vi "Ray2p0andDir.vi"(10 "Ray":T1) -> (2 "Dir":dbl[](array[numeric]), 3 "P0":dbl[](array[numeric]))   [LabVIEW 2014]
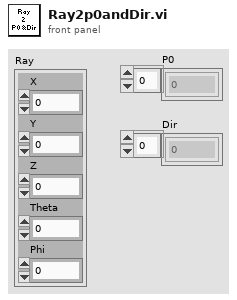
[diagram p1: front panel]
types:
  T1 = cluster{"X":dbl, "Y":dbl, "Z":dbl, "Theta":dbl, "Phi":dbl}
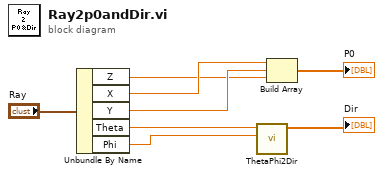
[diagram p0: block diagram]
diagram:
  n1 = Unbundle By Name("Ray") -> ("Z"=w1:dbl, "X"=w5:dbl, "Y"=w6:dbl, "Theta"=w3:dbl, "Phi"=w2:dbl)
  n2 = call "ThetaPhi2Dir.vi"("Phi"=w2, "Theta"=w3) -> ("Dir"=→"Dir":dbl[])  [unwired: 9 in]
  n3 = Build Array(w5, w6, w1) -> (→"P0":dbl[])
